vi "LoadImage(String-FileContent).vi"(1 "ImageFileContent":string, 5 "error in (no error)":errorcluster) -> (15 "ImageOut":refnum<k24>, 17 "ImageSize":cluster{"Width":i32, "Height":i32}, 19 "error out":errorcluster)   [LabVIEW 2020, in "LcPictureBox.lvclass"]
uses:
  LcPictureBox.lvclass
  System.Drawing
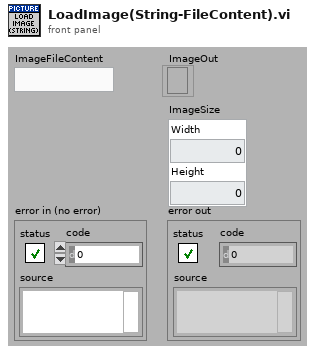
[diagram p1: front panel]
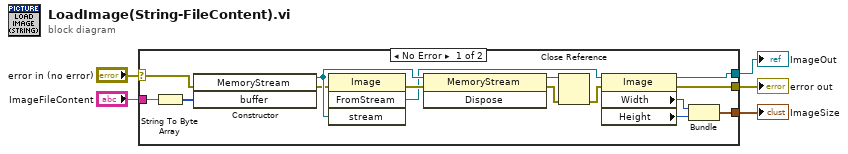
[diagram p0: block diagram]
diagram:
  n1 = case shown="No Error" "error in (no error)" {
    selector: "error in (no error)" -> [w9 w21]
    tunnel: [w19 w21] -> w4
    tunnel: "ImageFileContent" -> [w6 _]
    tunnel: [w20 _] -> w2
    tunnel: [w16 _] -> w1
    frame No Error {
      n2 = String To Byte Array(string=w6) -> (unsigned byte array=w10:u8[])
      n3 = constructor class="MemoryStream"(error in=w9, "buffer"=w10) -> (reference out=w15:refnum<k24>, error out=w11:errorcluster)  [unwired: 2 in, 2 out]
      n4 = invoke class="Image" method="FromStream"(error in=w11, "stream"=w15) -> (error out=w14:errorcluster, "FromStream"=w7:refnum<k24>)  [unwired: 2 in, 2 out]
      n5 = invoke class="MemoryStream" method="Dispose"(reference=w15, error in=w14) -> (reference out=w13:refnum<k24>, error out=w12:errorcluster)  [unwired: 1 in, 1 out]
      n6 = Close Reference(reference=w13, error in (no error)=w12) -> (error out=w8:errorcluster)
      n7 = property class="Image"(reference=w7, error in=w8) -> (reference out=w20:refnum<k24>, error out=w19:errorcluster, "Width"=w18:i32, "Height"=w17:i32)
      n8 = Bundle("Width"=w18, "Height"=w17) -> (w16:cluster{"Width":i32, "Height":i32})  [unwired: 1 in]
    }
    frame Error {
    }
  }
  "error out" <- w4
  "ImageOut" <- w2
  "ImageSize" <- w1
